vi "Intake_Execute.vi"() -> ()   [LabVIEW 2019]
uses:
  <vilib>/Rock Robotics/WPI/Solenoid/WPI_SolenoidValue.ctl
  Globals/Intake_Globals.vi
panel:
  out "Intake_Motor":dbl
  in  "Intake_Speed":dbl
  out "Intake_Extend":T1=enum."Reverse"
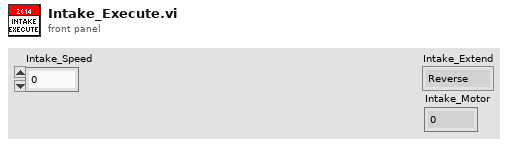
[diagram p1: front panel]
types:
  T1 = typedef "WPI_SolenoidValue.ctl" = enum16{"Off", "On", "Forward", "Reverse"}
  T2 = typedef "Intake_Cluster.ctl" = cluster{"Control_State":enum16{"Manual_Control"}, "Intake_On":bool, "Intake_Extended":bool}
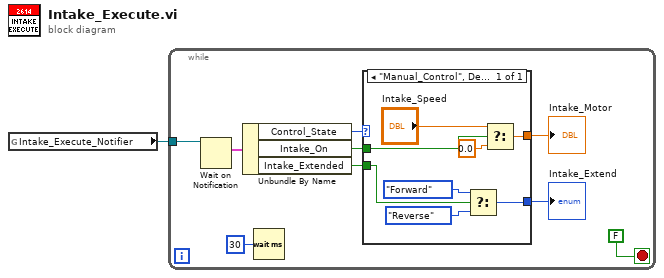
[diagram p0: block diagram]
diagram:
  n1 = global read "Intake_Globals.vi" "Intake_Execute_Notifier"() -> (w1:refnum<notifier>)
  n2 = while {
    tunnel: w1 -> [w9]
    stop <- FALSE stop-if-true
    n3 = Wait on Notification(notifier=w9) -> (notification=w8:T2)  [unwired: 3 in, 3 out]
    n4 = Unbundle By Name(w8) -> ("Control_State"=w7:enum16{"Manual_Control"}, "Intake_On"=w4:bool, "Intake_Extended"=w6:bool)
    n5 = Wait (ms)(milliseconds to wait=u32 30) -> ()  [unwired: 1 out]
    n6 = case shown="\"Manual_Control\", Default" w7 {
      tunnel: w6 -> [w17]
      tunnel: [w15] -> w5
      tunnel: w4 -> [w14]
      tunnel: [w11] -> w3
      frame "Manual_Control", Default {
        n7 = Select(t=WPI_SolenoidValue."Forward" ("Value"), s=w17, f=WPI_SolenoidValue."Reverse" ("Value")) -> (s? t:f=w15:T1)
        n8 = Select(t="Intake_Speed", s=w14, f=0.0) -> (s? t:f=w11:dbl)
      }
    }
    "Intake_Extend" <- w5
    "Intake_Motor" <- w3
  }
